vi "Main.vi"() -> ()   [LabVIEW 2018]
uses:
  typedefs/parttype.ctl
  typedefs/Machine state.ctl
  Diagnostic Message.ctl
  <vilib>/xnet/xnet.llb/XNET Database Close (Database).vi
panel:
  out "Flash Pass":bool
  in  "Read ECU Info":bool
  in  "Config Standard ECU Info":bool
  out "ECU Info OK":bool
  in  "Manual Print":bool
  in  "Parttype":T1
  in  "Start Flash":bool
  in  "Config ODX Path":bool
  out "ECU Info":T2
  out "CAL Time":dbl caption="CAL Time(s)" format="%.2f"
  out "Download CAL Progress":u8(slide) scale=0.0..100.0
  in  "Stop Button":bool
  out "error out":errorcluster
  in  "error in (no error)":errorcluster
  # "Version: 1.0"
  # "SCU Flash Station"
  # "Version 1.5"
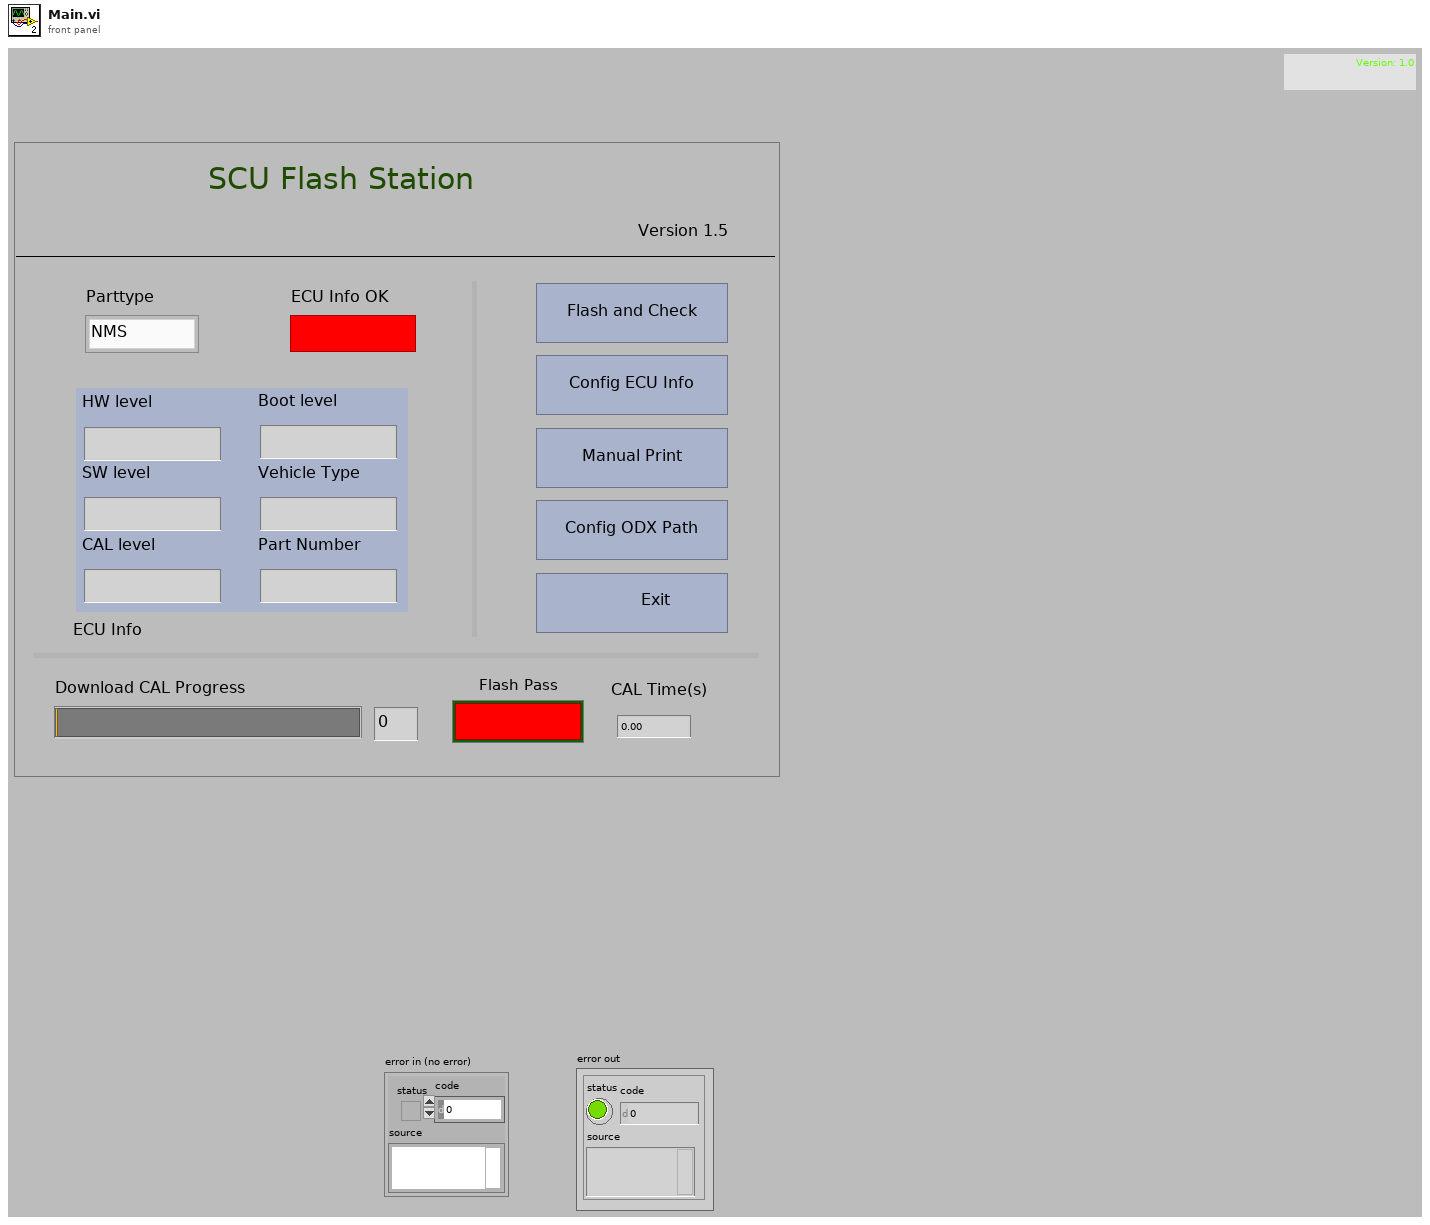
[diagram p1: front panel]
types:
  T1 = typedef "parttype.ctl" = enum16{"NMS", "B-SUV"}
  T2 = cluster{"HW level":string, "SW level":string, "CAL level":string, "Boot level":string, "Vehicle Type":string, "Part Number":string}
  T3 = enum16{"Query Device Info", "Set Voltage", "Read Voltage", "Set Current", "Read Current", "Enable Output", "Disable Output", "Set to Remote", "Set to Local", "Get Errors", "Set Protect Voltage", "Read Protect Voltage"}
  T4 = enum32{"invalid app kind", "Development System", "Run Time System", "Student Edition", "Embedded LabVIEW", "Evaluation", "Custom"}
  T5 = cluster{"ECU Info":cluster{"HW level":string, "SW level":string, "CAL level":string, "Boot level":string, "Vehicle Type":string, "Part Number":string}, "Manual Print":bool, "Parttype":T1, "SN":string, "autotest":bool}
  T6 = typedef "Machine state.ctl" = enum16{"Idle", "Config ODX path", "Update Standard ECU Info", "StartCAN", "Download ODX", "Read ECU Info", "StopCAN", "Manual Print", "Print label", "Save data", "Type"}
  T7 = typedef "Diagnostic Message.ctl" = enum16{"User Select", "Get User Multi-Frame", "Diag Session Prog", "Diag Session Ext", "Diag Session EOL", "Diag Session Default", "Diag Session Dev", "Read Active Session", "Read HW", "Read SW", "Read Part Number", "Learn Start Glass", "Learn Start Rollo", "Get Calibration Status", "Read SW CAL Boot", "Go to Position", "Get Parametric Mode Status", "Enable Parametric Mode", "Disable Parametric Mode", "Enable Production Mode", "Disable Production Mode", "Reset ECU", "Go to Slide Close", "Go to Slide Open", "Go to Vent Open", "Rollo Open", "Rollo Close", "Write Vehicle Type", "Read Vehicle Type", "Clear DTC", "Check Teach DTC", "Write Shop Code", "Download CAL", "Finish Flash", "Delete RP RF", "Download FBL"}
  T8 = typedef "barcode format params.ctl" = cluster{"Format String":string, "Print String":string, "Quantity":u8, "printer type":T9, "RS232 Port":string, "IP Address":string, "Ethernet Port":u32}
  T9 = typedef "barcode printer types.ctl" = enum16{"Intermec RS232", "Intermec Ethernet"}
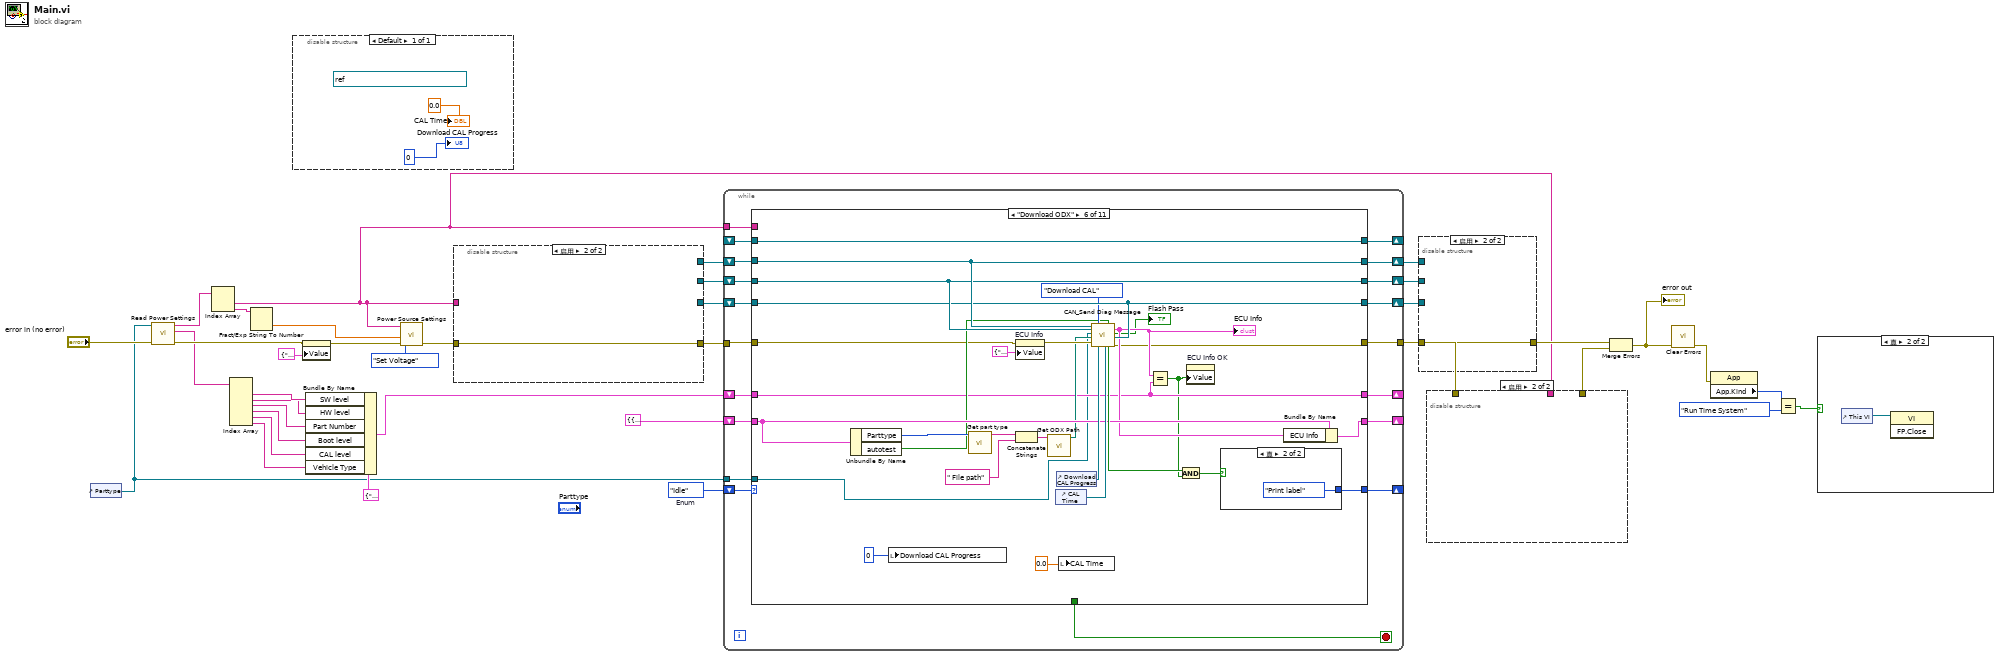
[diagram p0: block diagram]
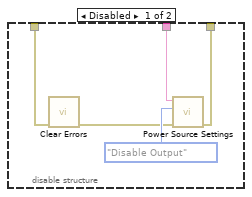
[diagram p3: hidden frame]
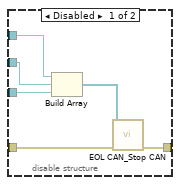
[diagram p4: hidden frame]
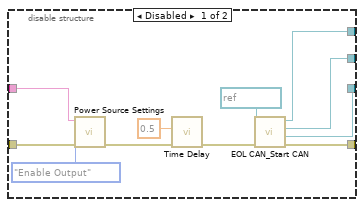
[diagram p5: hidden frame]
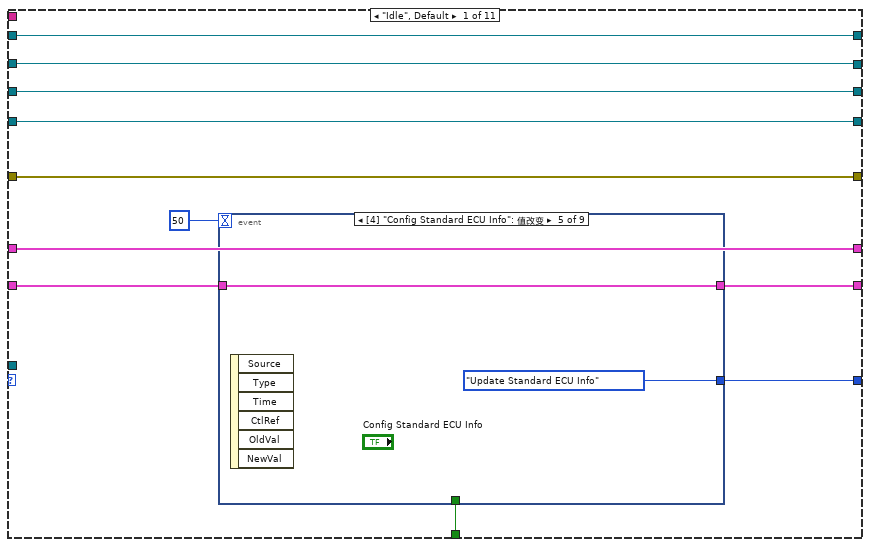
[diagram p6: hidden frame]
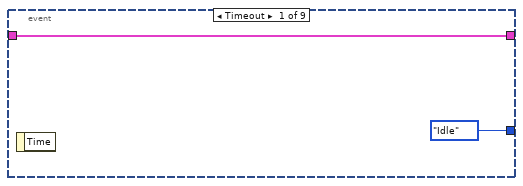
[diagram p7: hidden frame]
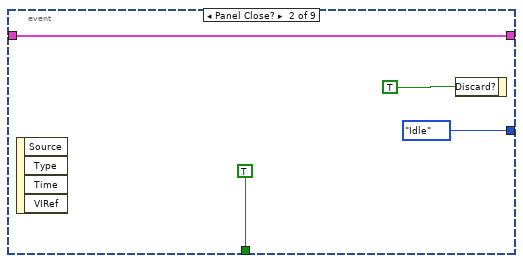
[diagram p8: hidden frame]
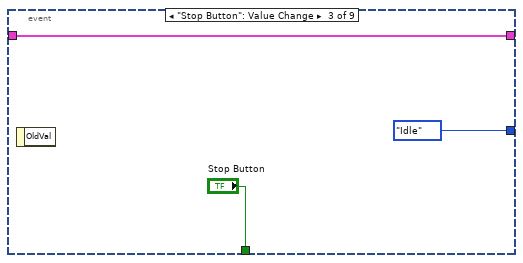
[diagram p9: hidden frame]
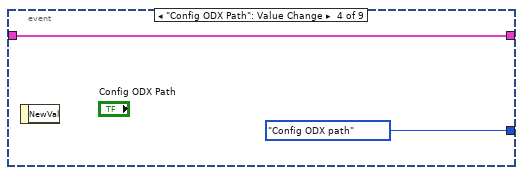
[diagram p10: hidden frame]
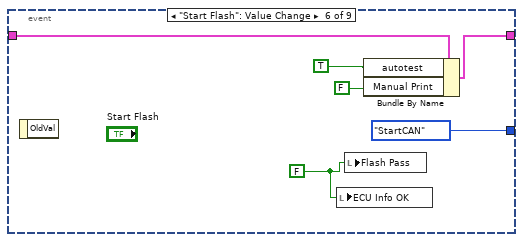
[diagram p11: hidden frame]
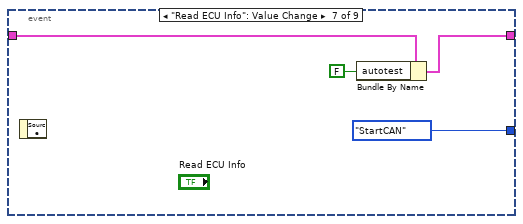
[diagram p12: hidden frame]
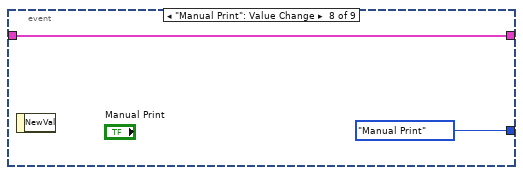
[diagram p13: hidden frame]
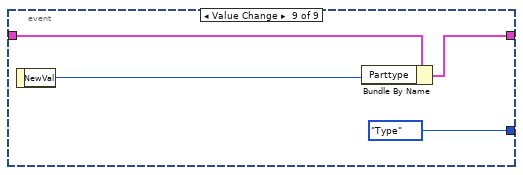
[diagram p14: hidden frame]
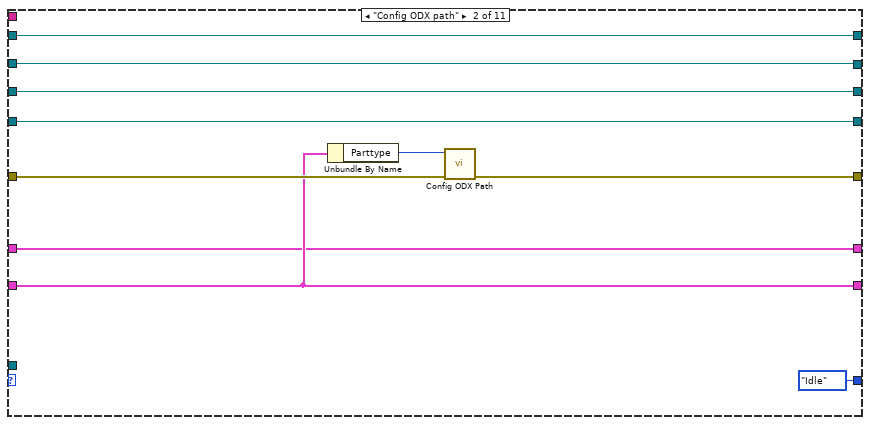
[diagram p15: hidden frame]
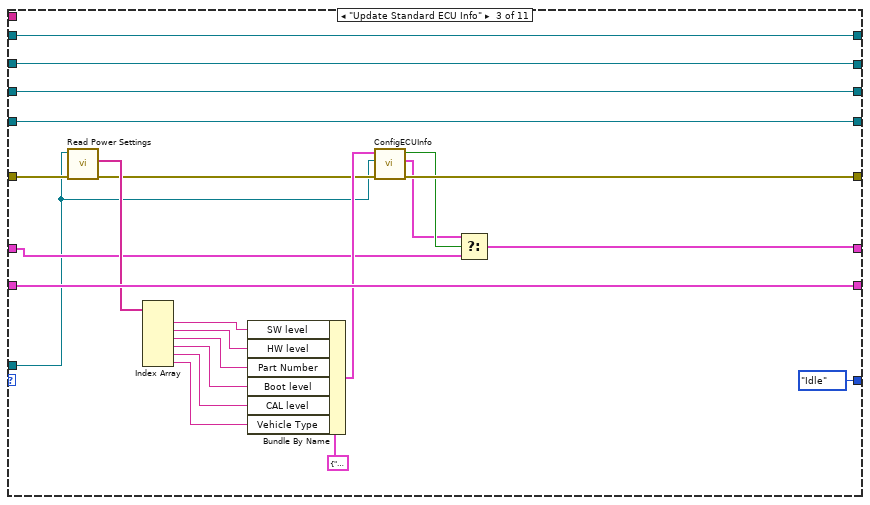
[diagram p16: hidden frame]
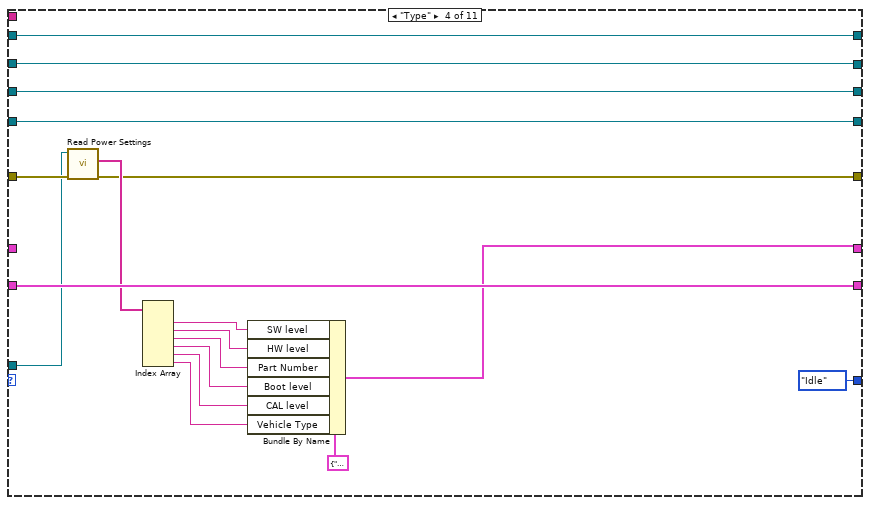
[diagram p17: hidden frame]
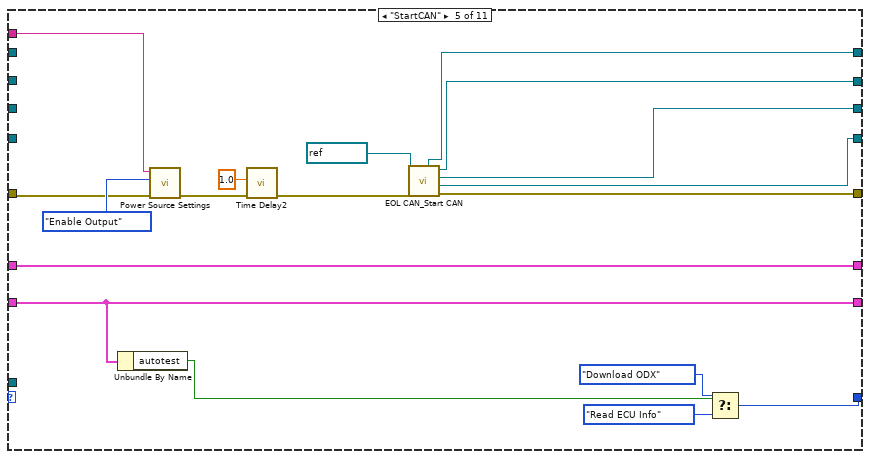
[diagram p18: hidden frame]
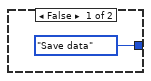
[diagram p19: hidden frame]
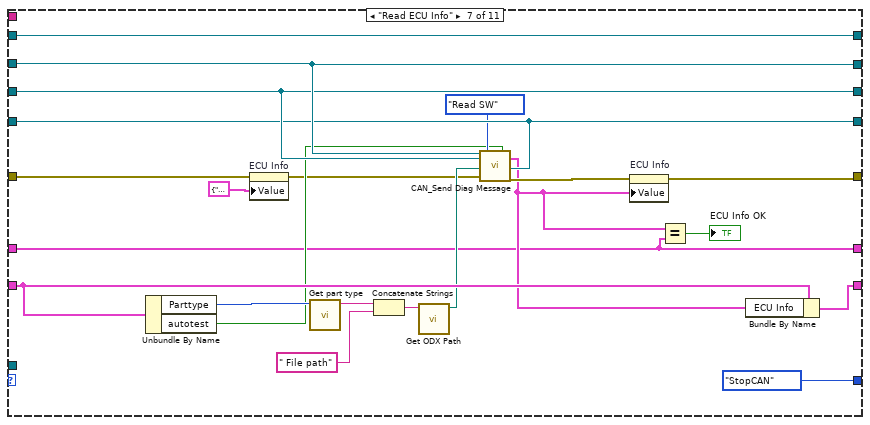
[diagram p20: hidden frame]
diagram:
  w27 = Machine_state."Idle"  # Enum
  n1 = control-ref of="Parttype"() -> (w2:refnum<vi>)
  n2 = call "Read Power Settings.vi"("error in (no error)"="error in (no error)", "Parttype"=w2) -> ("error out"=w21:errorcluster, "ECU Info"=w16:string[], "Power setting"=w20:string[])  [unwired: 7 in]
  n3 = Index Array(array=w20) -> (element #1=w8:string, element #2=w19:string)  [unwired: 2 in]
  n4 = Index Array(array=w16) -> (element #1=w15:string, element #2=w14:string, element #3=w13:string, element #4=w12:string, element #5=w11:string, element #6=w10:string)  [unwired: 6 in]
  n5 = Fract/Exp String To Number(string=w19) -> (number=w18:dbl)  [unwired: 3 in, 1 out]
  n6 = disable-structure shown="Default" {
    frame Enabled {
      (unwired) refnum<k21> "MLBevo_KCAN_KMatrix_V8" ("XNET Database")
      "CAL Time" <- 0.0 ("CAL Time")
      "Download CAL Progress" <- u8 0 ("Download CAL Progress")
    }
  }
  n7 = property on="ECU Info" class="Clust (严格)"(error in=w21, "Value"=T2 {"HW level"="", "SW level"="", "CAL level"="", "Boot level"="", "Vehicle Type"="", "Part Number"=""} ("ECU Info")) -> (error out=w26:errorcluster)  [unwired: 1 in, 1 out]
  n8 = Bundle By Name(cluster=T2 {"HW level"="", "SW level"="", "CAL level"="", "Boot level"="", "Vehicle Type"="", "Part Number"=""} ("ECU Info"), "SW level"=w15, "HW level"=w14, "Part Number"=w13, "Boot level"=w12, "CAL level"=w11, "Vehicle Type"=w10) -> (w9:T2)
  n9 = call "Power Source Settings.vi"("error in"=w26, "volt"=w18, "Action"=T3."Set Voltage", "COM"=w8) -> ("error out"=w28:errorcluster)  [unwired: 6 in, 1 out]
  n10 = disable-structure shown="启用" {
    disable-tunnel: [w50 w51] -> w36
    disable-tunnel: [w49 _] -> w35
    disable-tunnel: [w48 _] -> w34
    disable-tunnel: [w47 _] -> w31
    disable-tunnel: w28 -> [w45 w51]
    disable-tunnel: w8 -> [w41 _]
    frame Disabled {
      n11 = call "Power Source Settings.vi"("error in"=w45, "Action"=T3."Enable Output", "COM"=w41) -> ("error out"=w44:errorcluster)  [unwired: 7 in, 1 out]
      n12 = call "Time Delay"("error in (no error)"=w44, "Delay Time (s)"=0.5) -> ("error out"=w43:errorcluster)  [unwired: 9 in]
      n13 = call "EOL CAN_Start CAN.vi"("error in (no error)"=w43, "CAN Interface"=refnum<k21> "CAN1" ("CAN interface")) -> ("error out"=w50:errorcluster, "Tester Write Session out"=w48:refnum<k21>, "Read Session out"=w47:refnum<k21>, "DSC Write Session out"=w49:refnum<k21>)  [unwired: 5 in, 1 out]
    }
    frame Enabled {
    }
  }
  n14 = while {
    tunnel: w36 -> [w69]
    tunnel: [w70] -> w23
    shift-right: [w67] -> _
    shift-left: T5 {"ECU Info"={"HW level"="", "SW level"="", "CAL level"="", "Boot level"="", "Vehicle Type"="", "Part Number"=""}, "Manual Print"=FALSE, "Parttype"=enum."NMS", "SN"="", "autotest"=TRUE} -> [w65]
    shift-right: [w68] -> w37
    shift-left: w35 -> [w63]
    shift-right: [w66] -> w32
    shift-left: w31 -> [w64]
    shift-right: [w61] -> w33
    shift-left: w34 -> [w62]
    shift-right: [w59] -> _
    shift-left: w27 -> [w60]
    shift-right: [w57] -> _
    shift-left: w9 -> [w58]
    tunnel: w8 -> [w55]
    shift-right: [w54] -> _
    shift-left: _ -> [w53]
    tunnel: w2 -> [w52]
    stop <- w56 stop-if-true
    n15 = case shown="\"Download ODX\"" w60 {
      tunnel: [w80 w116 w126 w145 w178 w185 w212 w243 w260 w281 w288] -> w70
      tunnel: w69 -> [w80 w117 w138 w156 w171 w186 w213 w243 w264 w282 w302]
      tunnel: w63 -> [w81 w120 w143 w161 _ w208 w232 w246 w267 w285 w294]
      tunnel: [w81 w120 w143 w161 w177 w208 w232 w246 w267 w285 refnum<k21> refnum ("DSC Write Session out")] -> w68
      tunnel: w64 -> [w79 w119 w142 w160 _ w207 w231 w245 w266 w284 w293]
      tunnel: [w74 w115 w140 w158 w167 w198 w228 w235 w254 w276 w304] -> w67
      tunnel: [w79 w119 w142 w160 w176 w207 w231 w245 w266 w284 refnum<k21> refnum ("Read Session out")] -> w66
      tunnel: w65 -> [w75 w115 w140 w158 w167 w199 w229 w241 w257 w276 w304]
      tunnel: w62 -> [w78 w118 w141 w159 _ w204 w230 w244 w265 w283 w301]
      tunnel: [w78 w118 w141 w159 w175 w204 w230 w244 w265 w283 refnum<k21> refnum ("Tester Write Session out")] -> w61
      tunnel: [w76 Machine_state."Idle" ("Enum") Machine_state."Idle" ("Enum") Machine_state."Idle" ("Enum") w164 w200 Machine_state."StopCAN" ("Enum") w242 w251 Machine_state."StopCAN" ("Enum") Machine_state."Idle" ("Enum")] -> w59
      tunnel: w58 -> [w73 w112 w123 _ w168 w187 w215 w234 w252 w275 w305]
      tunnel: [w73 w112 w122 w144 w168 w187 w215 w234 w252 w275 w305] -> w57
      tunnel: [w72 _ _ _ _ _ _ _ _ _ _] -> w56
      tunnel: w55 -> [_ _ _ _ w170 _ _ _ _ _ w297]
      tunnel: [w71 w111 w129 w147 w162 w184 w211 w233 w250 w274 refnum<k21> refnum ("XNET Database")] -> w54
      tunnel: w53 -> [w71 w111 w129 w147 _ w184 w211 w233 w250 w274 w287]
      tunnel: w52 -> [_ _ w121 w146 _ w180 _ _ _ _ _]
      frame "Idle", Default {
        n16 = event shown="[4] \"Config Standard ECU Info\": 值改变" {
          selector: _ -> [_ _ _ _ _ _ _ _ _]
          dyn-events: _ -> [_ _ _ _ _ _ _ _ _]
          timeout: 50 -> [_ _ _ _ _ _ _ _ _]
          tunnel: [Machine_state."Idle" ("Enum") Machine_state."Idle" ("Enum") Machine_state."Idle" ("Enum") Machine_state."Config ODX path" ("Enum") Machine_state."Update Standard ECU Info" ("Enum") Machine_state."StartCAN" ("Enum") Machine_state."StartCAN" ("Enum") Machine_state."Manual Print" ("Enum") Machine_state."Type" ("Enum")] -> w76
          tunnel: w75 -> [w82 w85 w89 w91 w94 w98 w103 w105 w110]
          tunnel: [w82 w85 w89 w91 w94 w97 w102 w105 w108] -> w74
          tunnel: [_ TRUE ("Stop Button") "Stop Button" _ _ _ _ _ _] -> w72
          event Timeout {
            n17 = event-data() -> ()  [unwired: 1 in, 1 out]
          }
          event Panel Close? {
            n18 = event-data() -> ()  [unwired: 1 in, 4 out]
            n19 = event-data("Discard?"=TRUE) -> ()  [unwired: 1 in, 1 out]
          }
          event "Stop Button": Value Change {
            n20 = event-data() -> ()  [unwired: 1 in, 1 out]
          }
          event "Config ODX Path": Value Change {
            n21 = event-data() -> ()  [unwired: 1 in, 1 out]
          }
          event "Config Standard ECU Info": Value Change {
            n22 = event-data() -> ()  [unwired: 1 in, 6 out]
          }
          event "Start Flash": Value Change {
            w95 = FALSE ("Flash Fail")
            n23 = event-data() -> ()  [unwired: 1 in, 1 out]
            n24 = local write "ECU Info OK"(w95) -> ()
            n25 = local write "Flash Pass"(w95) -> ()
            n26 = Bundle By Name(cluster=w98, "autotest"=TRUE, "Manual Print"=FALSE) -> (w97:T5)
          }
          event "Read ECU Info": Value Change {
            n27 = event-data() -> ()  [unwired: 1 in, 1 out]
            n28 = Bundle By Name(cluster=w103, "autotest"=FALSE) -> (w102:T5)
          }
          event "Manual Print": Value Change {
            n29 = event-data() -> ()  [unwired: 1 in, 1 out]
          }
          event Value Change {
            n30 = event-data() -> ("NewVal"=w109:T1)  [unwired: 1 in]
            n31 = Bundle By Name(cluster=w110, "Parttype"=w109) -> (w108:T5)
          }
        }
      }
      frame "Config ODX path" {
        n32 = Unbundle By Name(w115) -> ("Parttype"=w114:T1)
        n33 = call "Config ODX Path.vi"("error in (no error)"=w117, "Parttype"=w114) -> ("error out"=w116:errorcluster)  [unwired: 9 in]
      }
      frame "Update Standard ECU Info" {
        n34 = call "Read Power Settings.vi"("error in (no error)"=w138, "Parttype"=w121) -> ("error out"=w127:errorcluster, "ECU Info"=w130:string[])  [unwired: 7 in, 1 out]
        n35 = Index Array(array=w130) -> (element #1=w132:string, element #2=w133:string, element #3=w134:string, element #4=w135:string, element #5=w136:string, element #6=w137:string)  [unwired: 6 in]
        n36 = Bundle By Name(cluster=T2 {"HW level"="", "SW level"="", "CAL level"="", "Boot level"="", "Vehicle Type"="", "Part Number"=""} ("ECU Info"), "SW level"=w132, "HW level"=w133, "Part Number"=w134, "Boot level"=w135, "CAL level"=w136, "Vehicle Type"=w137) -> (w128:T2)
        n37 = call "ConfigECUInfo.vi"("error in (no error)"=w127, "Parttype"=w121, "ECU Info"=w128) -> ("error out"=w126:errorcluster, "ECU Info"=w124:T2, "change?"=w125:bool)  [unwired: 6 in]
        n38 = Select(t=w124, s=w125, f=w123) -> (s? t:f=w122:T2)
      }
      frame "Type" {
        n39 = call "Read Power Settings.vi"("error in (no error)"=w156, "Parttype"=w146) -> ("error out"=w145:errorcluster, "ECU Info"=w148:string[])  [unwired: 7 in, 1 out]
        n40 = Index Array(array=w148) -> (element #1=w150:string, element #2=w151:string, element #3=w152:string, element #4=w153:string, element #5=w154:string, element #6=w155:string)  [unwired: 6 in]
        n41 = Bundle By Name(cluster=T2 {"HW level"="", "SW level"="", "CAL level"="", "Boot level"="", "Vehicle Type"="", "Part Number"=""} ("ECU Info"), "SW level"=w150, "HW level"=w151, "Part Number"=w152, "Boot level"=w153, "CAL level"=w154, "Vehicle Type"=w155) -> (w144:T2)
      }
      frame "StartCAN" {
        n42 = Unbundle By Name(w167) -> ("autotest"=w166:bool)
        n43 = call "Power Source Settings.vi"("error in"=w171, "Action"=T3."Enable Output", "COM"=w170) -> ("error out"=w172:errorcluster)  [unwired: 7 in, 1 out]
        n44 = call "Time Delay2"("error in (no error)"=w172, "Delay Time (s)"=1.0) -> ("error out"=w169:errorcluster)  [unwired: 9 in]
        n45 = call "EOL CAN_Start CAN.vi"("error in (no error)"=w169, "CAN Interface"=refnum<k21> "CAN1" ("CAN interface")) -> ("error out"=w178:errorcluster, "Tester Write Session out"=w175:refnum<k21>, "Read Session out"=w176:refnum<k21>, "DSC Write Session out"=w177:refnum<k21>, "XNET Database"=w162:refnum<k21>)  [unwired: 5 in]
        n46 = Select(t=Machine_state."Download ODX" ("Enum"), s=w166, f=Machine_state."Read ECU Info") -> (s? t:f=w164:T6)
      }
      frame "Download ODX" {
        n47 = Unbundle By Name(w199) -> ("Parttype"=w196:T1, "autotest"=w189:bool)
        n48 = local write "Download CAL Progress"(u8 0 ("Download CAL Progress")) -> ()
        n49 = call "Get part type.vi"("Enum"=w196) -> ("Parttype"=w195:string)  [unwired: 10 in]
        n50 = Concatenate Strings(w195, " File path" ("string")) -> (w193:string)
        n51 = property on="ECU Info" class="Clust (严格)"(error in=w186, "Value"=T2 {"HW level"="", "SW level"="", "CAL level"="", "Boot level"="", "Vehicle Type"="", "Part Number"=""} ("ECU Info")) -> (error out=w203:errorcluster)  [unwired: 1 in, 1 out]
        n52 = call "Get ODX Path.vi"("ODX type"=w193) -> ("Current Path"=w197:path)  [unwired: 9 in, 1 out]
        n53 = control-ref of="CAL Time"() -> (w205:refnum<vi>)
        n54 = control-ref of="Download CAL Progress"() -> (w206:refnum<vi>)
        n55 = local write "CAL Time"(0.0 ("CAL Time")) -> ()
        n56 = call "CAN_Send Diag Message.vi"("Write Session in"=w208, "Read Session in"=w207, "Parttype ref"=w180, "ODX File Path"=w197, "error in (no error)"=w203, "Enum"=Diagnostic_Message."Download CAL", "Download CAL Progress"=w206, "Download CAL Time"=w205, "Autotest"=w189, "Tester"=w204) -> ("Response Good?"=w201:bool, "ECU Info"=w188:T2, "pass?"=→"Flash Pass":bool, "error out"=w185:errorcluster)  [unwired: 5 in, 1 out]
        "ECU Info" <- w188
        n57 = Equal?(x=w188, y=w187) -> (x = y?=w182:bool)
        n58 = And(x=w201, y=w182) -> (x .and. y?=w183:bool)
        n59 = property on="ECU Info OK" class="Bool (严格)"("Value"=w182) -> ()  [unwired: 2 in, 2 out]
        n60 = case shown="真" w183 {
          tunnel: [Machine_state."Save data" ("Enum") Machine_state."Print label" ("Enum")] -> w200
          frame False {
          }
          frame True {
          }
        }
        n61 = Bundle By Name(cluster=w199, "ECU Info"=w188) -> (w198:T5)
      }
      frame "Read ECU Info" {
        n62 = Unbundle By Name(w229) -> ("Parttype"=w226:T1, "autotest"=w221:bool)
        n63 = property on="ECU Info" class="Clust (严格)"(error in=w213, "Value"=T2 {"HW level"="", "SW level"="", "CAL level"="", "Boot level"="", "Vehicle Type"="", "Part Number"=""} ("ECU Info")) -> (error out=w220:errorcluster)  [unwired: 1 in, 1 out]
        n64 = call "Get part type.vi"("Enum"=w226) -> ("Parttype"=w225:string)  [unwired: 10 in]
        n65 = Concatenate Strings(w225, " File path" ("string")) -> (w223:string)
        n66 = call "Get ODX Path.vi"("ODX type"=w223) -> ("Current Path"=w227:path)  [unwired: 9 in, 1 out]
        n67 = call "CAN_Send Diag Message.vi"("Write Session in"=w232, "Read Session in"=w231, "ODX File Path"=w227, "error in (no error)"=w220, "Enum"=Diagnostic_Message."Read SW", "Autotest"=w221, "Tester"=w230) -> ("ECU Info"=w216:T2, "error out"=w217:errorcluster)  [unwired: 8 in, 3 out]
        n68 = property on="ECU Info" class="Clust (严格)"(error in=w217, "Value"=w216) -> (error out=w212:errorcluster)  [unwired: 1 in, 1 out]
        n69 = Equal?(x=w216, y=w215) -> (x = y?=→"ECU Info OK":bool)
        n70 = Bundle By Name(cluster=w229, "ECU Info"=w216) -> (w228:T5)
      }
      frame "Manual Print" {
        n71 = call "Manual print UI.vi"() -> ("Print?"=w237:bool, "ECU Info"=w238:T2, "Parttype"=w239:T1, "SN"=w240:string)  [unwired: 8 in]
        n72 = Bundle By Name(cluster=w241, "Manual Print"=TRUE, "SN"=w240, "Parttype"=w239, "ECU Info"=w238) -> (w235:T5)
        n73 = case shown="真" w237 {
          tunnel: [Machine_state."Idle" ("Enum") Machine_state."Print label" ("Enum")] -> w242
          frame False {
          }
          frame True {
          }
        }
      }
      frame "Print label" {
        n74 = Unbundle By Name(w257) -> ("ECU Info"=w261:T2, "Parttype"=w259:T1, "SN"=w253:string, "Manual Print"=w255:bool)
        n75 = call "Get part type.vi"("Enum"=w259) -> ("Parttype"=w258:string)  [unwired: 10 in]
        n76 = call "read barcode formats.vi"("error in"=w264) -> ("error out"=w263:errorcluster, "Frame Barcode Formats"=w262:T8[])  [unwired: 9 in]
        n77 = call "Barcode Print.vi"("SN"=w253, "Manual?"=w255, "error in"=w263, "ECU Info"=w261, "Frame Barcode Formats"=w262, "part type"=w258) -> ("error out"=w260:errorcluster, "SN out"=w249:string)  [unwired: 4 in]
        n78 = case shown="真" w255 {
          tunnel: [w268 w272] -> w256
          tunnel: w253 -> [_ w271]
          tunnel: [Machine_state."Save data" ("Enum") Machine_state."Idle" ("Enum")] -> w251
          tunnel: w249 -> [w268 _]
          frame False {
          }
          frame True {
            n79 = Concatenate Strings("M" ("string"), w271) -> (w272:string)
          }
        }
        n80 = Bundle By Name(cluster=w257, "SN"=w256) -> (w254:T5)
      }
      frame "Save data" {
        n81 = Unbundle By Name(w276) -> ("ECU Info"=w280:T2, "SN"=w279:string, "Parttype"=w278:T1)
        n82 = call "Save test data.vi"("error in"=w282, "Parttype"=w278, "SN"=w279, "ECU Info"=w280) -> ("error out"=w281:errorcluster)  [unwired: 7 in]
      }
      frame "StopCAN" {
        n83 = Build Array(w294, w293, w301) -> (w303:refnum<k21>[])
        n84 = call "EOL CAN_Stop CAN.vi"("error in (no error)"=w302, "XNET Session Array In"=w303) -> ("error out"=w298:errorcluster)  [unwired: 9 in]
        n85 = call "Time Delay3"("error in (no error)"=w298, "Delay Time (s)"=0.2) -> ("error out"=w296:errorcluster)  [unwired: 9 in]
        n86 = call "Power Source Settings.vi"("error in"=w296, "Action"=T3."Disable Output", "COM"=w297) -> ("error out"=w289:errorcluster)  [unwired: 7 in, 1 out]
        n87 = call-poly <vilib>:"XNET Database Close.vi"("database in"=w287, "error in (no error)"=w289) -> ("error out"=w288:errorcluster)  [unwired: 13 in]
      }
    }
  }
  n88 = disable-structure shown="启用" {
    disable-tunnel: w37 -> [w310 _]
    disable-tunnel: w33 -> [w309 _]
    disable-tunnel: w32 -> [w308 _]
    disable-tunnel: [w307 w312] -> w24
    disable-tunnel: w23 -> [w306 w312]
    frame Disabled {
      n89 = Build Array(w310, w308, w309) -> (w311:refnum<k21>[])
      n90 = call "EOL CAN_Stop CAN.vi"("error in (no error)"=w306, "XNET Session Array In"=w311) -> ("error out"=w307:errorcluster)  [unwired: 9 in]
    }
    frame Enabled {
    }
  }
  n91 = disable-structure shown="启用" {
    disable-tunnel: w23 -> [w316 _]
    disable-tunnel: [w314 _] -> w22
    disable-tunnel: w8 -> [w313 _]
    frame Disabled {
      n92 = call <vilib>:"Clear Errors.vi"("error in (no error)"=w316) -> ("error out"=w315:errorcluster)  [unwired: 5 in, 1 out]
      n93 = call "Power Source Settings.vi"("error in"=w315, "Action"=T3."Disable Output", "COM"=w313) -> ("error out"=w314:errorcluster)  [unwired: 7 in, 1 out]
    }
    frame Enabled {
    }
  }
  n94 = Merge Errors(w24, w22) -> (w4:errorcluster)
  "error out" <- w4
  n95 = call <vilib>:"Clear Errors.vi"("error in (no error)"=w4) -> ("error out"=w5:errorcluster)  [unwired: 5 in, 1 out]
  n96 = property class="App"(error in=w5) -> ("App.Kind"=w6:T4)  [unwired: 1 in, 2 out]
  n97 = Equal?(x=w6, y=T4."Run Time System" ("Application:Kind")) -> (x = y?=w3:bool)
  n98 = case shown="真" w3 {
    frame False {
    }
    frame True {
      n99 = control-ref of="This VI"() -> (w318:refnum<vi>)
      n100 = invoke class="VI" method="FP.Close"(reference=w318) -> ()  [unwired: 2 in, 3 out]
    }
  }
